vi "slink query energy.vi"(8 "error in (no error)":errorcluster, 10 "# channels":i32, 11 "VISA Refnum in":refnum<visa-resource-name>) -> (0 "error out":errorcluster, 1 "Channel 2 value":dbl, 2 "Channel 1 value":dbl, 3 "VISA Refnum out":refnum<visa-resource-name>, 5 "String":string)   [LabVIEW 2020]
uses:
  Gentec Slink.lvclass
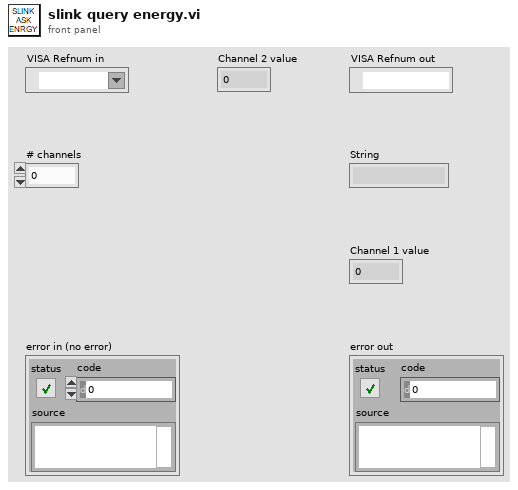
[diagram p1: front panel]
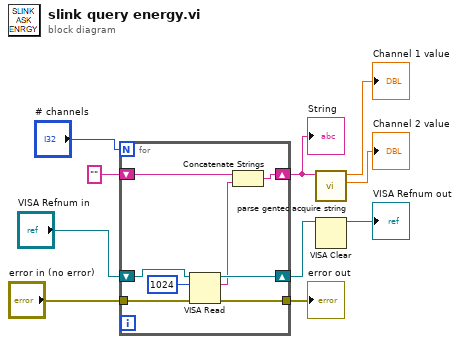
[diagram p0: block diagram]
diagram:
  n1 = for {
    N: "# channels" -> [_]
    tunnel: [w15] -> w2
    shift-right: [w17] -> w8
    shift-left: "VISA Refnum in" -> [w18]
    shift-right: [w13] -> w3
    shift-left: "" -> [w12]
    tunnel: "error in (no error)" -> [w11]
    n2 = VISA Read(VISA resource name=w18, byte count=u32 1024, error in (no error)=w11) -> (VISA resource name out=w17:refnum<visa-resource-name>, read buffer=w14:string, error out=w15:errorcluster)  [unwired: 1 out]
    n3 = Concatenate Strings(w12, w14) -> (w13:string)
  }
  "String" <- w3
  "error out" <- w2
  n4 = call "parse gentec acquire string.vi"("Acquisition String"=w3) -> ("Channel 2 value"=→"Channel 2 value":dbl, "Channel 1 value"=→"Channel 1 value":dbl)  [unwired: 9 in]
  n5 = VISA Clear(VISA resource name=w8) -> (VISA resource name out=→"VISA Refnum out":refnum<visa-resource-name>)  [unwired: 1 in, 1 out]
